vi "check numeric validity.vi"(2 "Numeric string":string) -> (7 "Valid ?":bool)   [LabVIEW 2020]
doc: "The purpose of this VI is to check whether the incoming string is numeric (INT or FLOAT) or not.\nThe incoming string should be in the form of numbers only - no short forms or engineering units (k, E, M etc are allowed)"
panel:
  out "after substring":string
  out "match substring":string
  out "before substring":string
  out "offset past match":i32
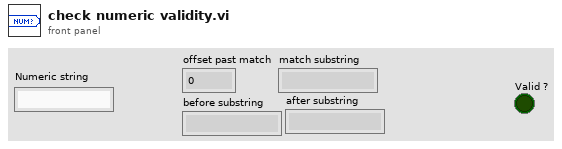
[diagram p1: front panel]
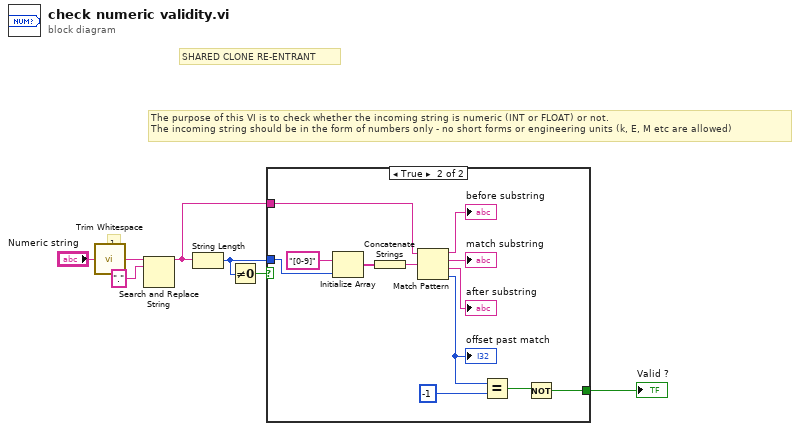
[diagram p0: block diagram]
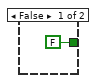
[diagram p2: hidden frame]
diagram:
  # "SHARED CLONE RE-ENTRANT"
  # "The purpose of this VI is to check whether the incoming string is numeric (INT or FLOAT) or not.\nThe incoming string should be in the form of numbers only - no short forms or engineering units (k, E, M etc are allowed)"
  # "1."
  n1 = call <vilib>:"Trim Whitespace.vi"("string"="Numeric string") -> ("trimmed string"=w3:string)  [unwired: 1 in]
  n2 = Search and Replace String(input string=w3, search string=".") -> (result string=w1:string)  [unwired: 6 in, 3 out]
  n3 = String Length(string=w1) -> (length=w7:i32)
  n4 = Not Equal To 0?(x=w7) -> (x != 0?=w6:bool)
  n5 = case shown="True" w6 {
    tunnel: w7 -> [_ w20]
    tunnel: w1 -> [_ w16]
    tunnel: [FALSE w9] -> w4
    frame False {
    }
    frame True {
      n6 = Initialize Array("[0-9]", w20) -> (w18:string[])
      n7 = Concatenate Strings(w18) -> (w17:string)
      n8 = Match Pattern(string=w16, regular expression=w17) -> (before substring=→"before substring":string, match substring=→"match substring":string, after substring=→"after substring":string, offset past match=w12:i32)  [unwired: 1 in]
      "offset past match" <- w12
      n9 = Equal?(x=w12, y=-1) -> (x = y?=w10:bool)
      n10 = Not(x=w10) -> (.not. x?=w9:bool)
    }
  }
  "Valid ?" <- w4
